vi "CSV Reader.vi"(6 "Reset":bool, 7 "Index in":i32, 10 "Parcel Length":i32, 11 "Config":T2={"Mode"=enum."Full timestamp", "delimiter (\\t)"="\t", "Path"=path "", "Rectangular?"=FALSE}) -> (1 "Analog":dbl[][](array[numeric]), 2 "Complex":cdb[][](array[numeric]), 3 "Timestamps":timestamp[](array[timestamp]), 4 "EOF?":bool, 5 "Index out":i32)   [LabVIEW 2017]
uses:
  Mode CSV reader.ctl
  <vilib>/Utility/file.llb/Read Delimited Spreadsheet (DBL).vi
  <vilib>/Utility/file.llb/Read Delimited Spreadsheet (string).vi
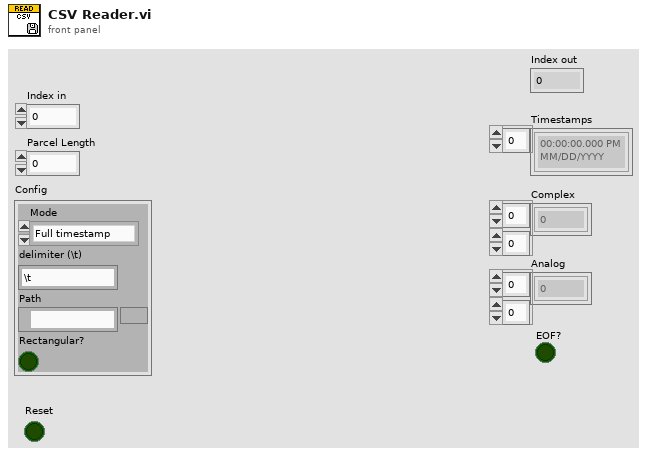
[diagram p1: front panel]
types:
  T1 = typedef "Mode CSV reader.ctl" = enum16{"Full timestamp", "Relative Time", "Seconds Time", "Nanoseconds Time"}
  T2 = cluster{"Mode":T1, "delimiter (\\t)":string, "Path":path, "Rectangular?":bool}
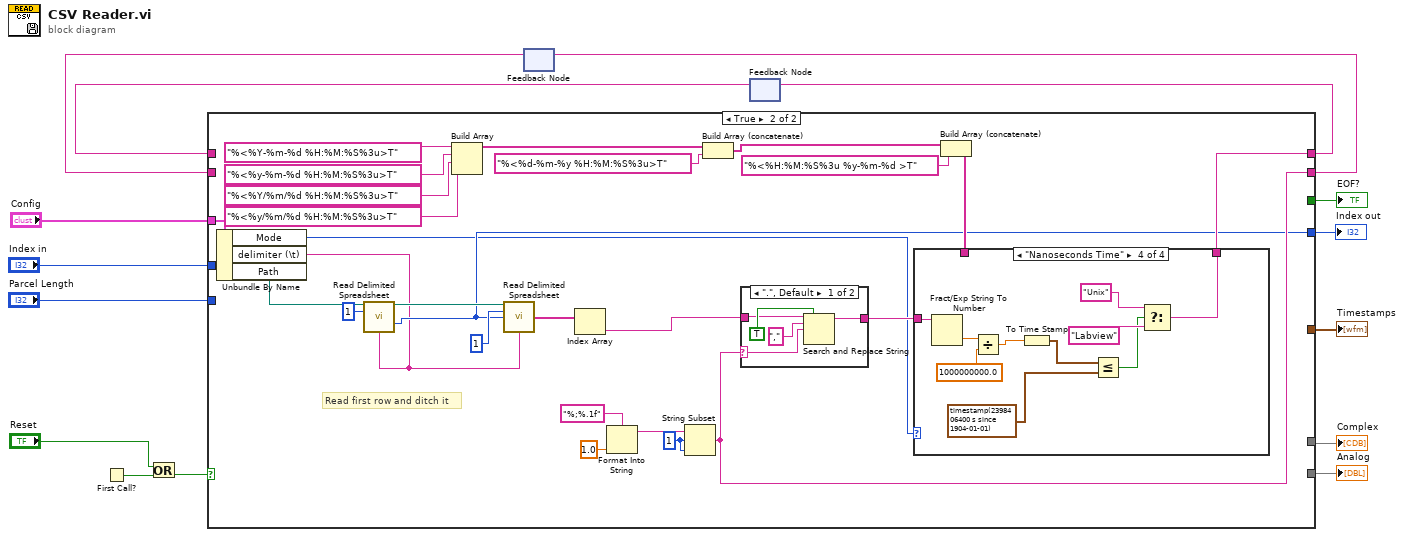
[diagram p0: block diagram]
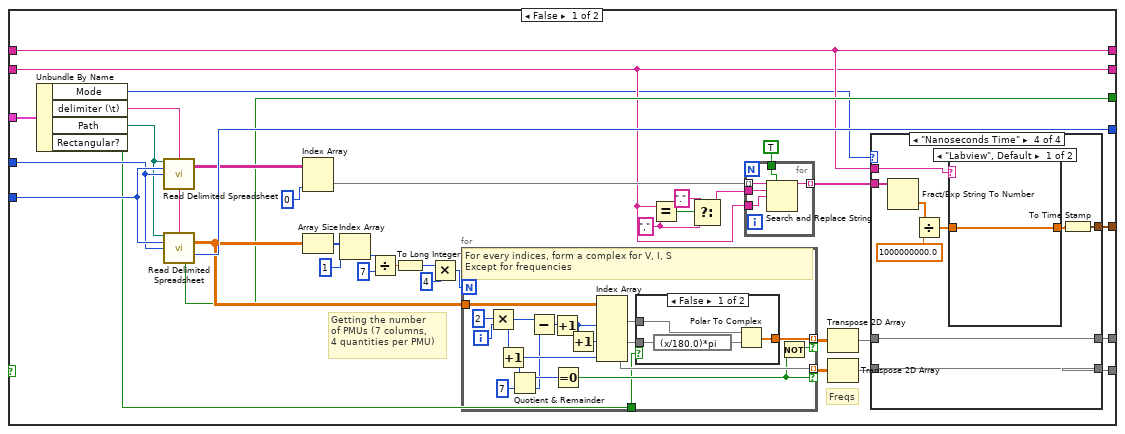
[diagram p2: hidden frame]
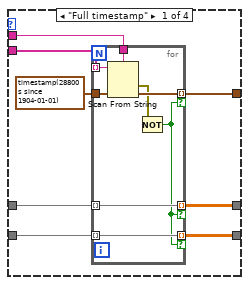
[diagram p3: hidden frame]
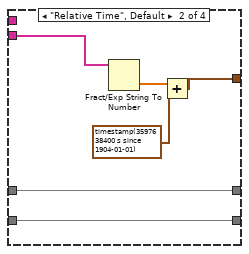
[diagram p4: hidden frame]
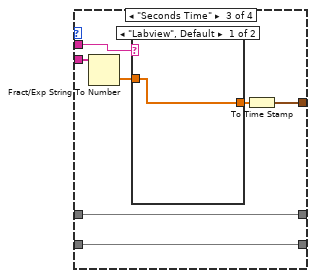
[diagram p5: hidden frame]
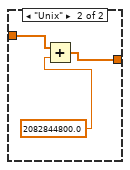
[diagram p6: hidden frame]
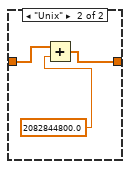
[diagram p7: hidden frame]
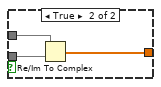
[diagram p8: hidden frame]
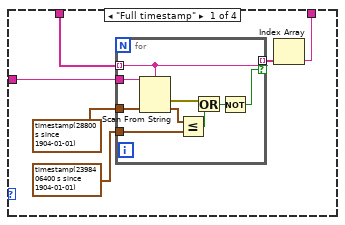
[diagram p9: hidden frame]
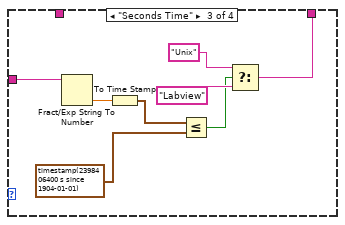
[diagram p11: hidden frame]
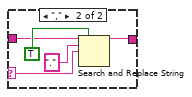
[diagram p12: hidden frame]
diagram:
  n1 = First Call?() -> (First Call?: T/F=w15:bool)
  n2 = Or(x="Reset", y=w15) -> (x .or. y?=w4:bool)
  n3 = feedback #1() -> (w11:string)  [unwired: 1 in]
  n4 = feedback #2() -> (w13:string)  [unwired: 1 in]
  n5 = case shown="True" w4 {
    tunnel: [w35 w145] -> w14
    tunnel: w13 -> [w35 _]
    tunnel: [w27 w135] -> w12
    tunnel: w11 -> [w27 _]
    tunnel: [w49 w132] -> w10
    tunnel: "Index in" -> [w50 _]
    tunnel: "Parcel Length" -> [w51 _]
    tunnel: [w39 _] -> w7
    tunnel: [w36 _] -> w6
    tunnel: "Config" -> [w26 w131]
    tunnel: [w21 _] -> w1
    tunnel: [w20 _] -> w2
    frame False {
      w29 = "," ("search string")
      # "Freqs"
      # "Getting the number\nof PMUs (7 columns, \n4 quantities per PMU)"
      n6 = Unbundle By Name(w26) -> ("Mode"=w25:T1, "delimiter (\\t)"=w24:string, "Path"=w23:path, "Rectangular?"=w22:bool)
      n7 = call-poly <vilib>:"Read Delimited Spreadsheet.vi"("file path (dialog if empty)"=w23, "number of rows (all:-1)"=w51, "start of read offset (chars.:0)"=w50, "delimiter (\\t)"=w24) -> ("all rows"=w38:string[][])  [unwired: 6 in, 5 out]
      n8 = call-poly <vilib>:"Read Delimited Spreadsheet.vi"("file path (dialog if empty)"=w23, "number of rows (all:-1)"=w51, "start of read offset (chars.:0)"=w50, "delimiter (\\t)"=w24) -> ("all rows"=w40:dbl[][], "mark after read (chars.)"=w49:i32, "EOF?"=w36:bool)  [unwired: 6 in, 3 out]
      n9 = Index Array(array=w38, index (col)=0 ("disabled index (col)")) -> (element=w34:string[])  [unwired: 1 in]
      n10 = Array Size(array=w40) -> (size(s)=w43:i32[])
      n11 = Index Array(array=w43, index=1) -> (element=w45:i32)
      n12 = Divide(x=w45, y=7) -> (x/y=w47:dbl)
      n13 = To Long Integer(number=w47) -> (32bit integer=w41:i32)
      n14 = Multiply(x=w41, y=4) -> (x*y=w42:i32)
      n15 = for {
        N: w42 -> [_]
        tunnel: [w118] -> w19 mode=indexing if=w108
        tunnel: w40 -> [w115]
        tunnel: [w109] -> w18 mode=indexing if=w107
        tunnel: w22 -> [w103]
        i -> [w111]
        # "For every indices, form a complex for V, I, S\nExcept for frequencies"
        n16 = Multiply(x=2, y=w111) -> (x*y=w104:i32)
        n17 = Increment(x=w104) -> (x+1=w110:i32)
        n18 = Quotient & Remainder(x=w110, y=7) -> (x-y*floor(x/y)=w112:i32, floor(x/y)=w105:i32)
        n19 = Subtract(x=w104, y=w105) -> (x-y=w106:i32)
        n20 = Increment(x=w106) -> (x+1=w116:i32)
        n21 = Equal To 0?(x=w112) -> (x = 0?=w107:bool)
        n22 = Increment(x=w116) -> (x+1=w114:i32)
        n23 = Index Array(array=w115, index (col) #1=w116, index (col) #2=w114, index (col) #3=w110) -> (element #1=w119:dbl[], element #2=w120:dbl[], element #3=w109:dbl[])  [unwired: 3 in]
        n24 = case shown="False" w103 {
          tunnel: w120 -> [w123 w127]
          tunnel: w119 -> [w122 w126]
          tunnel: [w124 w125] -> w118
          frame False {
            n25 = expression code="(x/180.0)*pi" ("degrees to radians")(w123) -> (w121:dbl[])
            n26 = Polar To Complex(1:w121, 2:w122) -> (0:w124:cdb[])
          }
          frame True {
            n27 = Re/Im To Complex(1:w127, 2:w126) -> (0:w125:cdb[])
          }
        }
        n28 = Not(x=w107) -> (.not. x?=w108:bool)
      }
      n29 = Equal?(x=w27, y=w29) -> (x = y?=w28:bool)
      n30 = Select(t="." ("search string"), s=w28, f=w29) -> (s? t:f=w30:string)
      n31 = for {
        tunnel: w34 -> [w56] mode=indexing
        tunnel: [w55] -> w33 mode=indexing
        tunnel: w27 -> [w53]
        tunnel: TRUE ("replace all? (F)") -> [w54]
        tunnel: w30 -> [w52]
        n32 = Search and Replace String(replace all?=w54, input string=w56, search string=w52, replace string=w53) -> (result string=w55:string)  [unwired: 4 in, 3 out]
      }
      n33 = Transpose 2D Array(2D array=w19) -> (transposed array=w17:cdb[][])
      n34 = Transpose 2D Array(2D array=w18) -> (transposed array=w16:dbl[][])
      n35 = case shown="\"Nanoseconds Time\"" w25 {
        tunnel: [w63 w77 w84 w97] -> w39
        tunnel: w33 -> [w62 w76 w85 w98]
        tunnel: w35 -> [w61 _ w81 w90]
        tunnel: w17 -> [w60 w74 w83 w94]
        tunnel: w16 -> [w59 w73 w82 w93]
        tunnel: [w58 w74 w83 w94] -> w21
        tunnel: [w57 w73 w82 w93] -> w20
        frame "Full timestamp" {
          n36 = for {
            tunnel: w61 -> [w72]
            tunnel: timestamp(28800 s since 1904-01-01) ("default value 1") -> [w71]
            tunnel: [w70] -> w63 mode=indexing if=w65
            tunnel: w62 -> [w69] mode=indexing
            tunnel: w60 -> [w68] mode=indexing
            tunnel: w59 -> [w67] mode=indexing
            tunnel: [w68] -> w58 mode=indexing if=w65
            tunnel: [w67] -> w57 mode=indexing if=w65
            n37 = Scan From String(format string=w72, input string=w69, default 1=w71) -> (error out=w66:errorcluster, output 1=w70:timestamp)  [unwired: 2 in, 2 out]
            n38 = Not(x=w66) -> (.not. x?=w65:bool)
          }
        }
        frame "Relative Time", Default {
          n39 = Fract/Exp String To Number(string=w76) -> (number=w75:dbl[])  [unwired: 3 in, 1 out]
          n40 = Add(x=w75, y=timestamp(3597638400 s since 1904-01-01) ("default value 1")) -> (x+y=w77:timestamp[])
        }
        frame "Seconds Time" {
          n41 = Fract/Exp String To Number(string=w85) -> (number=w80:dbl[])  [unwired: 3 in, 1 out]
          n42 = case shown="\"Labview\", Default" w81 {
            tunnel: w80 -> [w86 w89]
            tunnel: [w86 w87] -> w79
            frame "Labview", Default {
            }
            frame "Unix" {
              n43 = Add(x=w89, y=2082844800.0 ("x-y")) -> (x+y=w87:dbl[])
            }
          }
          n44 = To Time Stamp(1:w79) -> (0:w84:timestamp[])
        }
        frame "Nanoseconds Time" {
          n45 = Fract/Exp String To Number(string=w98) -> (number=w96:dbl[])  [unwired: 3 in, 1 out]
          n46 = Divide(x=w96, y=1000000000.0 ("result string")) -> (x/y=w92:dbl[])
          n47 = case shown="\"Labview\", Default" w90 {
            tunnel: [w99 w101] -> w91
            tunnel: w92 -> [w99 w100]
            frame "Labview", Default {
            }
            frame "Unix" {
              n48 = Add(x=w100, y=2082844800.0 ("x-y")) -> (x+y=w101:dbl[])
            }
          }
          n49 = To Time Stamp(1:w91) -> (0:w97:timestamp[])
        }
      }
    }
    frame True {
      w136 = 1 ("offset (0)")
      # "Read first row and ditch it"
      n50 = Unbundle By Name(w131) -> ("Mode"=w130:T1, "delimiter (\\t)"=w128:string, "Path"=w129:path)
      n51 = call-poly <vilib>:"Read Delimited Spreadsheet.vi"("file path (dialog if empty)"=w129, "number of rows (all:-1)"=1, "delimiter (\\t)"=w128) -> ("new file path (Not A Path if cancelled)"=w147:path, "mark after read (chars.)"=w132:i32)  [unwired: 7 in, 4 out]
      n52 = Build Array("%<%Y-%m-%d %H:%M:%S%3u>T", "%<%y-%m-%d %H:%M:%S%3u>T", "%<%Y/%m/%d %H:%M:%S%3u>T", "%<%y/%m/%d %H:%M:%S%3u>T") -> (w144:string[])
      n53 = call-poly <vilib>:"Read Delimited Spreadsheet.vi"("file path (dialog if empty)"=w147, "number of rows (all:-1)"=1, "start of read offset (chars.:0)"=w132, "delimiter (\\t)"=w128) -> ("first row"=w146:string[])  [unwired: 6 in, 5 out]
      n54 = Index Array(array=w146) -> (element=w133:string)  [unwired: 1 in]
      n55 = Format Into String(format string="%;%.1f", 1.0 ("input 1")) -> (resulting string=w137:string)  [unwired: 2 in, 1 out]
      n56 = String Subset(string=w137, offset (0)=w136, length (rest)=w136) -> (substring=w135:string)
      n57 = Build Array (concatenate)(w144, "%<%d-%m-%y %H:%M:%S%3u>T") -> (w142:string[])
      n58 = case shown="\".\", Default" w135 {
        selector: w135 -> [w189 w193]
        tunnel: [w191 w194] -> w134
        tunnel: w133 -> [w187 w192]
        frame ".", Default {
          n59 = Search and Replace String(replace all?=TRUE ("replace all? (F)"), input string=w187, search string=",", replace string=w189) -> (result string=w191:string)  [unwired: 4 in, 3 out]
        }
        frame "," {
          n60 = Search and Replace String(replace all?=TRUE ("replace all? (F)"), input string=w192, search string=".", replace string=w193) -> (result string=w194:string)  [unwired: 4 in, 3 out]
        }
      }
      n61 = Build Array (concatenate)(w142, "%<%H:%M:%S%3u %y-%m-%d >T") -> (w140:string[])
      n62 = case shown="\"Nanoseconds Time\"" w130 {
        tunnel: [w158 _ w172 w177] -> w145
        tunnel: w140 -> [w157 _ _ _]
        tunnel: w134 -> [w156 _ w175 w181]
        frame "Full timestamp" {
          n63 = for {
            tunnel: w157 -> [w164] mode=indexing
            tunnel: timestamp(2398406400 s since 1904-01-01) ("default value 1") -> [w168]
            tunnel: [w164] -> w155 mode=indexing if=w161
            tunnel: w156 -> [w163]
            tunnel: timestamp(28800 s since 1904-01-01) ("default value 1") -> [w160]
            n64 = Scan From String(format string=w164, input string=w163, default 1=w160) -> (error out=w167:errorcluster, output 1=w162:timestamp)  [unwired: 2 in, 2 out]
            n65 = Less Or Equal?(x=w162, y=w168) -> (x <= y?=w166:bool)
            n66 = Or(x=w167, y=w166) -> (x .or. y?=w165:bool)
            n67 = Not(x=w165) -> (.not. x?=w161:bool)
          }
          n68 = Index Array(array=w155) -> (element=w158:string)  [unwired: 1 in]
        }
        frame "Relative Time", Default {
        }
        frame "Seconds Time" {
          n69 = Fract/Exp String To Number(string=w175) -> (number=w174:dbl)  [unwired: 3 in, 1 out]
          n70 = To Time Stamp(1:w174) -> (0:w173:timestamp)
          n71 = Less Or Equal?(x=w173, y=timestamp(2398406400 s since 1904-01-01) ("default value 1")) -> (x <= y?=w169:bool)
          n72 = Select(t="Unix" ("result string"), s=w169, f="Labview" ("result string")) -> (s? t:f=w172:string)
        }
        frame "Nanoseconds Time" {
          n73 = Fract/Exp String To Number(string=w181) -> (number=w180:dbl)  [unwired: 3 in, 1 out]
          n74 = Divide(x=w180, y=1000000000.0) -> (x/y=w179:dbl)
          n75 = To Time Stamp(1:w179) -> (0:w185:timestamp)
          n76 = Less Or Equal?(x=w185, y=timestamp(2398406400 s since 1904-01-01) ("default value 1")) -> (x <= y?=w182:bool)
          n77 = Select(t="Unix" ("result string"), s=w182, f="Labview" ("result string")) -> (s? t:f=w177:string)
        }
      }
    }
  }
  "Index out" <- w10
  "Timestamps" <- w7
  "Complex" <- w1
  "Analog" <- w2
  "EOF?" <- w6
  n78 = feedback-in #1(w12) -> ()
  n79 = feedback-in #2(w14) -> ()
